vi "Graph ERD Read List.vi"(0 "GEA2 Reference In":refnum<k24>, 5 "GEA Inputs":T15={"Source"=229, "Destination"=35} {"Destination" format="%.0x"; "Source" format="%.0x"}, 7 "All_Bundled_Data_In":T1, 9 "ERD Graph Cntrl":T16={"ERD 3"={"ERD #"=0, "Data Type"=enum."uint16_t", "Scaler"=1}, "ERD 2"={"ERD #"=0, "Data Type"=enum."uint16_t", "Scaler"=1}, "ERD 1, ERD 2, & ERD3"={"ERD #"=0, "Data Type"=enum."uint16_t", "Scaler"=1}} {"ERD 1, ERD 2, & ERD3"."Scaler" min=1; "ERD 1, ERD 2, & ERD3"."ERD #" format="%.0x"; "ERD 2"."Scaler" min=1; "ERD 2"."ERD #" format="%.0x"; "ERD 3"."Scaler" min=1; "ERD 3"."ERD #" format="%.0x"}, 11 "Error In":errorcluster) -> (4 "GEA2 Reference Out":refnum<k24>, 6 "ERD Graph  Ind":T14, 10 "All_Bundled_Data_Brass Out":T1, 15 "Error Out":errorcluster)   [LabVIEW 2021]
uses:
  type defs/ERD_Graph_All_3.ctl
  type defs/ERD_Graph.ctl
  Common/LabVIEW GEA2 Toolkit/GEA3/type defs/Data Type.ctl
  D:/Common/LabVIEW GEA2 Toolkit/source/GEA3 DLL Source/GeaCommunication.dll
  Common/LabVIEW GEA2 Toolkit/source/GEA3 DLL Source/GeaCommunication.dll
  Common/LabVIEW GEA2 Toolkit/GEA3/type defs/Source_Destination.ctl
  type defs/All_Bundled_Data.ctl
  type defs/Version.ctl
  type defs/ERD_Always_Show.ctl
  type defs/Brass Matrix.ctl
  type defs/CSV_File_String_Arrays.ctl
  type defs/Redundant.ctl
  type defs/Algorithms.ctl
  type defs/ATC_Data.ctl
  type defs/Fault Table Array.ctl
  type defs/Fault_Table_Info.ctl
  Dryer Tool (Commercial 2)/JL Dryer Tool Support/type defs/ERD_RJ45.ctl
  Dryer Tool (Commercial 2)/JL Dryer Tool Support/type defs/ERD_Commercial_Laundry.ctl
  type defs/BootloaderVersion.ctl
  Common/LabVIEW GEA2 Toolkit/GEA3/type defs/ERD Read Data In.ctl
panel:
  # "Wet Load Size"
  # "Dry Load Size"
  # "OOB"
  # "Wet Load Size"
  # "Dry Load Size"
  # "OOB"
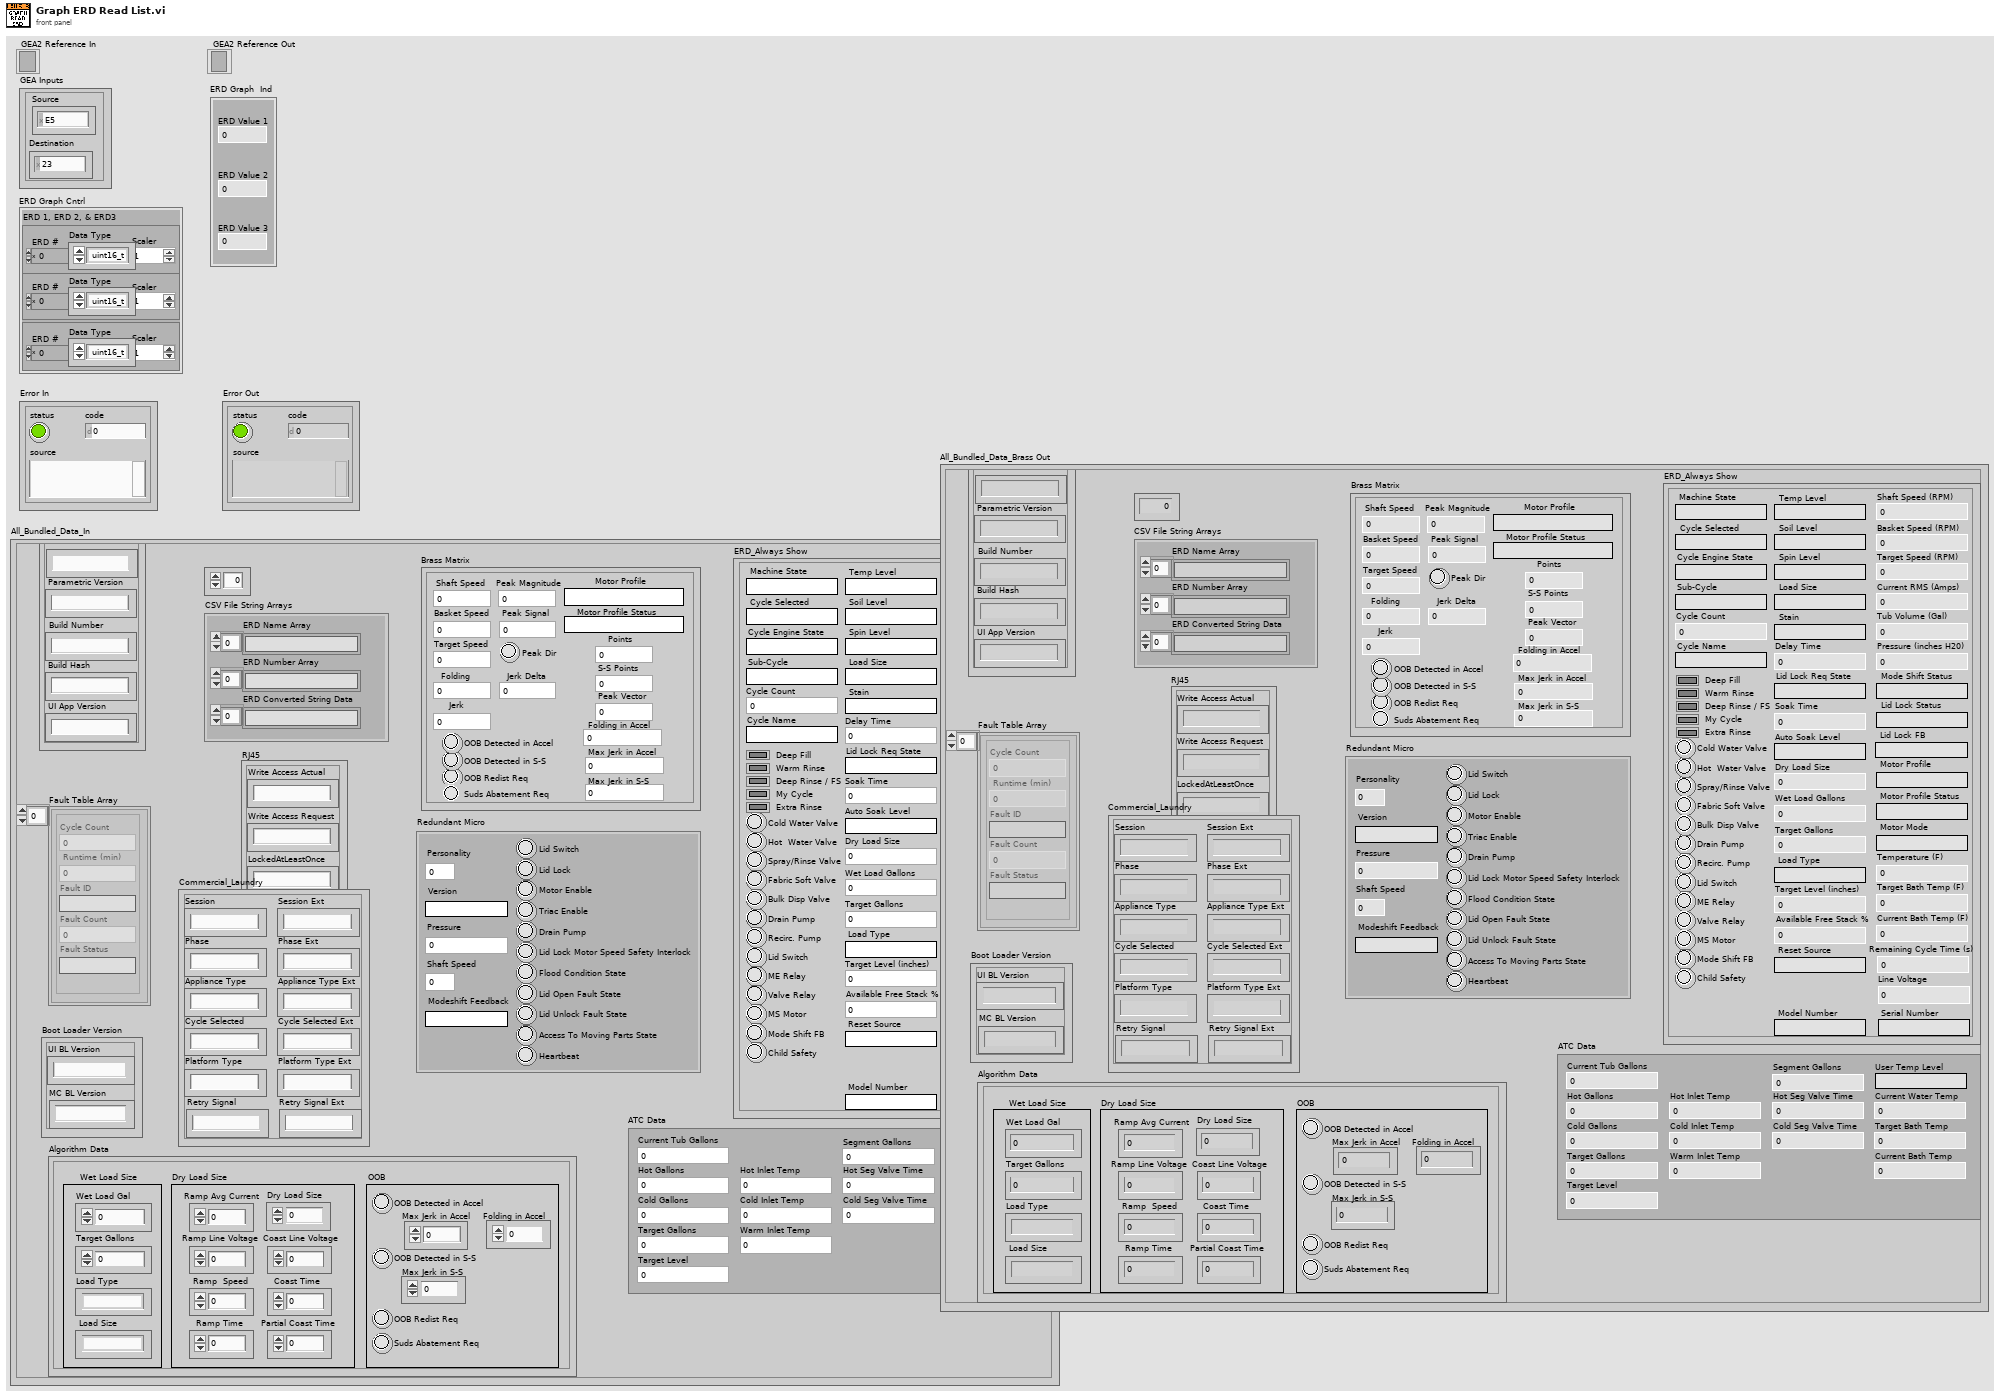
[diagram p1: front panel]
types:
  T1 = typedef "All_Bundled_Data.ctl" = cluster{"Software MC":T2, "ERD_Always Show":T3, "Personality Set":u8, "Brass Matrix":T4, "CSV File String Arrays":T5, "Redundant Micro":T6, "Algorithm Data":T7, "ATC Data":T8, "Fault Table Array ":T9, "RJ45":T11, "Commercial_Laundry":T12, "Boot Loader Version":T13}
  T2 = typedef "Version.ctl" = cluster{"Build Number":string, "Build Hash ":string, "Application Version":string, "Parametric Version":string, "UI App Version":string}
  T3 = typedef "ERD_Always_Show.ctl" = cluster{"Basket Speed (RPM)":u16, "Machine State":string, "Tub Volume (Gal)":dbl, "Pressure (inches H20)":dbl, "Lid Switch ":bool, "Current RMS (Amps)":dbl, "Cycle Selected":string, "Lid Lock Status":string, "Mode Shift Status":string, "Spray/Rinse Valve":bool, "Fabric Soft Valve":bool, "Drain Pump":bool, "Recirc. Pump":bool, "Cycle Engine State":string, "Hot  Water Valve":bool, "Cold Water Valve":bool, "Motor Profile":string, "Motor Profile Status":string, "Motor Mode":string, "ME Relay":bool, "Cycle Count":u32, "Deep Rinse / FS":bool, "My Cycle":bool, "Soil Level":string, "Spin Level":string, "Stain":string, "Temp Level":string, "Load Size":string, "Delay Time":u16, "Soak Time":u16, "Deep Fill":bool, "Warm Rinse":bool, "Auto Soak Level":string, "Extra Rinse":bool, "Wet Load Gallons":dbl, "Target Gallons":dbl, "Sub-Cycle":string, "Load Type":string, "Target Level (inches)":dbl, "Valve Relay":bool, "Dry Load Size":dbl, "Shaft Speed (RPM) ":u16, "MS Motor":bool, "Mode Shift FB":bool, "Target Bath Temp (F)":dbl, "Temperature (F)":dbl, "Current Bath Temp (F)":dbl, "Lid Lock FB":string, "Lid Lock Req State":string, "Remaining Cycle Time (s)":u32, "Available Free Stack %":u8, "Child Safety":bool, "Target Speed (RPM)":u16, "Reset Source":string, "Line Voltage":dbl, "Cycle Name":string, "Bulk Disp Valve":bool, "Model Number":string, "Serial Number":string}
  T4 = typedef "Brass Matrix.ctl" = cluster{"Shaft Speed":u16, "Folding":i32, "Jerk":i32, "Basket Speed":u16, "Target Speed":u16, "Peak Signal":u8, " Peak Magnitude":dbl, "Folding in Accel":i32, "Max Jerk in Accel":i32, "Max Jerk in S-S":i32, "Motor Profile Status":string, "Motor Profile":string, "OOB Redist Req":bool, "OOB Detected in S-S":bool, "OOB Detected in Accel":bool, "Suds Abatement Req ":bool, "Peak Dir":bool, "Peak Vector":dbl, "S-S Points":u8, "Points":u8, "Jerk Delta":i32}
  T5 = typedef "CSV_File_String_Arrays.ctl" = cluster{"ERD Number Array":string[], "ERD Name Array":string[], "ERD Converted String Data":string[]}
  T6 = typedef "Redundant.ctl" = cluster{"Version":string, "Personality":u8, "Pressure ":dbl, "Shaft Speed":u16, "Modeshift Feedback":string, "Lid Switch":bool, "Lid Lock":bool, "Triac Enable":bool, "Drain Pump":bool, "Lid Lock Motor Speed Safety Interlock":bool, "Flood Condition State":bool, "Lid Open Fault State":bool, "Access To Moving Parts State":bool, "Heartbeat":bool, "Motor Enable":bool, "Lid Unlock Fault State":bool}
  T7 = typedef "Algorithms.ctl" = cluster{"Wet Load Gal":dbl, "Target Gallons":dbl, "Load Type":string, "Load Size":string, "Coast Time":u16, "Ramp Time":u16, "Ramp  Speed":u16, "Ramp Avg Current":dbl, "OOB Redist Req":bool, "OOB Detected in S-S":bool, "Folding in Accel":i32, "Max Jerk in Accel":i32, "Max Jerk in S-S":i32, "OOB Detected in Accel":bool, "Partial Coast Time":u16, "Dry Load Size":dbl, "Ramp Line Voltage ":dbl, "Coast Line Voltage":dbl, "Suds Abatement Req ":bool}
  T8 = typedef "ATC_Data.ctl" = cluster{"Current Tub Gallons":dbl, "Hot Gallons":dbl, "Cold Gallons":dbl, "Target Gallons":dbl, "Current Water Temp":dbl, "Target Level":dbl, "Target Bath Temp":dbl, "Current Bath Temp ":dbl, "Cold Inlet Temp":dbl, "Hot Inlet Temp":dbl, "Warm Inlet Temp":dbl, "Hot Seg Valve Time":u16, "Cold Seg Valve Time ":u16, "User Temp Level":string, "Segment Gallons":dbl}
  T9 = typedef "Fault Table Array.ctl" = T10[]
  T10 = typedef "Fault_Table_Info.ctl" = cluster{"Cycle Count":u32, " Runtime (min) ":u32, "Fault Status":string, "Fault ID":string, "Fault Count":u16}
  T11 = typedef "ERD_RJ45.ctl" = cluster{"Write Access Actual":string, "Write Access Request":string, "LockedAtLeastOnce":string}
  T12 = typedef "ERD_Commercial_Laundry.ctl" = cluster{"Session":string, "Phase":string, "Appliance Type":string, "Cycle Selected":string, "Platform Type":string, "Retry Signal":string, "Session Ext":string, "Phase Ext":string, "Appliance Type Ext":string, "Cycle Selected Ext":string, "Platform Type Ext":string, "Retry Signal Ext":string}
  T13 = typedef "BootloaderVersion.ctl" = cluster{"UI BL Version":string, "MC BL Version":string}
  T14 = cluster{"ERD Value 1":dbl, "ERD Value 2":dbl, "ERD Value 3":dbl}
  T15 = typedef "Source_Destination.ctl" = cluster{"Source":u8, "Destination":u8}
  T16 = typedef "ERD_Graph_All_3.ctl" = cluster{"ERD 3":T17, "ERD 2":T17, "ERD 1, ERD 2, & ERD3":T17}
  T17 = typedef "ERD_Graph.ctl" = cluster{"ERD #":u16, "Data Type":T18, "Scaler":u32}
  T18 = typedef "Data Type.ctl" = enum16{"string", "boolean", "uint8_t", "uint16_t", "uint32_t", "uint64_t", "int8_t", "int16_t", "int32_t", "int64_t"}
  T19 = typedef "ERD Read Data In.ctl" = cluster{"ERD Number":u16, "Data Type":enum16{"string", "boolean", "uint8_t", "uint16_t", "uint32_t", "uint64_t", "int8_t", "int16_t", "int32_t", "int64_t"}}
  T20 = typedef "ERD Read Data Out.ctl" = cluster{"ERD Number":u16, "Data":string}
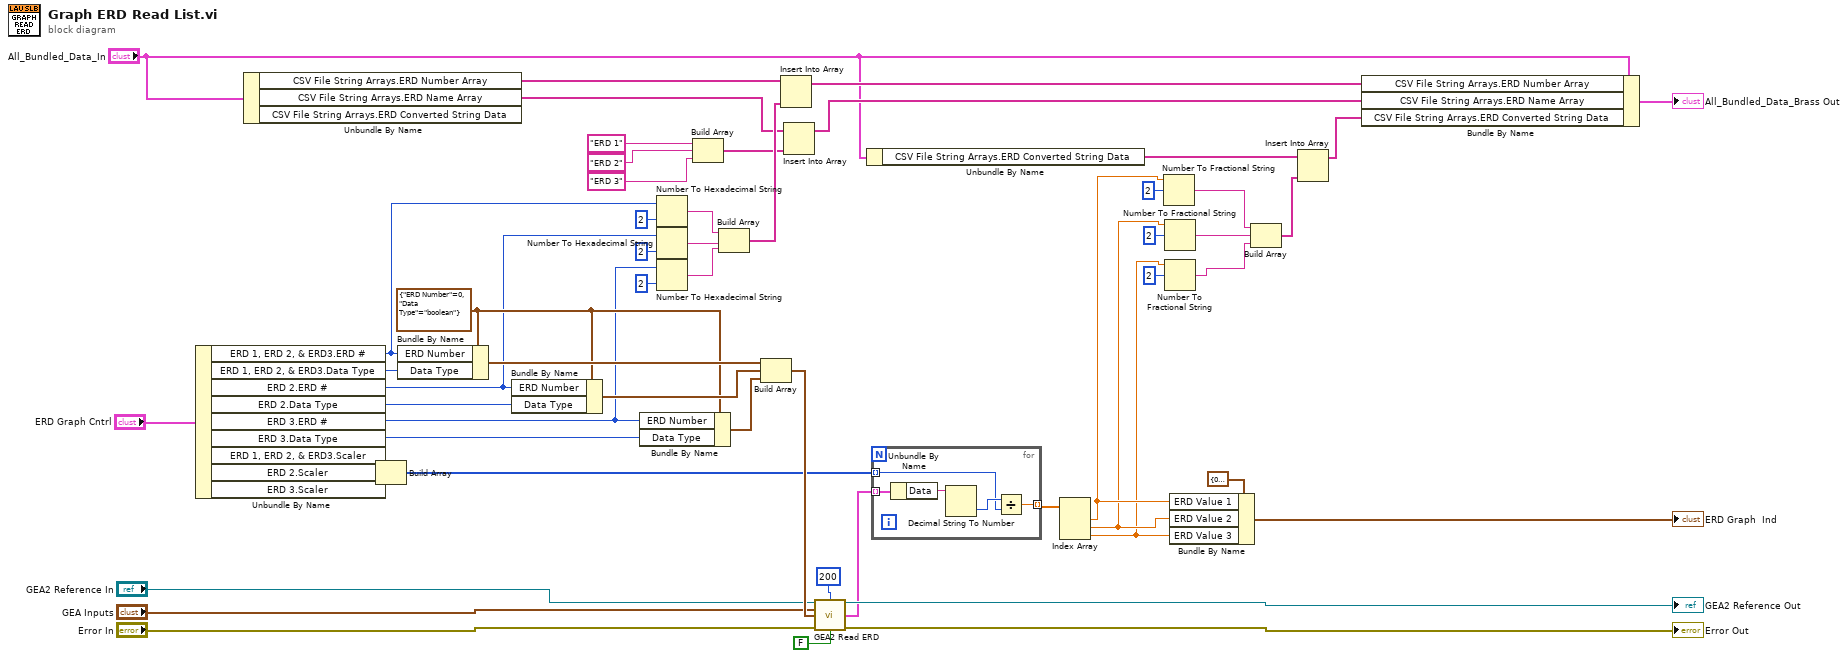
[diagram p0: block diagram]
diagram:
  w52 = T19 {"ERD Number"=0, "Data Type"=enum."boolean"} ("ERD Read Data In 2")
  n1 = Unbundle By Name("ERD Graph Cntrl") -> ("ERD 1, ERD 2, & ERD3.ERD #"=w29:u16, "ERD 1, ERD 2, & ERD3.Data Type"=w49:T18, "ERD 2.ERD #"=w28:u16, "ERD 2.Data Type"=w50:T18, "ERD 3.ERD #"=w27:u16, "ERD 3.Data Type"=w51:T18, "ERD 1, ERD 2, & ERD3.Scaler"=w42:u32, "ERD 2.Scaler"=w41:u32, "ERD 3.Scaler"=w40:u32)
  n2 = Unbundle By Name("All_Bundled_Data_In") -> ("CSV File String Arrays.ERD Number Array"=w22:string[], "CSV File String Arrays.ERD Name Array"=w19:string[])  [unwired: 1 out]
  n3 = Build Array(w42, w41, w40) -> (w39:u32[])
  n4 = Bundle By Name(cluster=w52, "ERD Number"=w29, "Data Type"=w49) -> (w53:T19)
  n5 = Bundle By Name(cluster=w52, "ERD Number"=w28, "Data Type"=w50) -> (w54:T19)
  n6 = Bundle By Name(cluster=w52, "ERD Number"=w27, "Data Type"=w51) -> (w55:T19)
  n7 = Number To Hexadecimal String(1:i16 2 ("width (-)"), 2:w29) -> (0:w26:string)
  n8 = Number To Hexadecimal String(1:i16 2 ("width (-)"), 2:w28) -> (0:w25:string)
  n9 = Number To Hexadecimal String(1:i16 2 ("width (-)"), 2:w27) -> (0:w24:string)
  n10 = Build Array("ERD 1", "ERD 2", "ERD 3") -> (w18:string[])
  n11 = Build Array(w26, w25, w24) -> (w23:string[])
  n12 = Build Array(w53, w54, w55) -> (w48:T19[])
  n13 = Insert Into Array(array=w22, new element=w23) -> (w20:string[])  [unwired: 1 in]
  n14 = Insert Into Array(array=w19, new element=w18) -> (w14:string[])  [unwired: 1 in]
  n15 = call "GEA2 Read ERD.vi"("GEA2 Reference In"="GEA2 Reference In", "Read Timeout (ms)"=u32 200, "GEA Inputs"="GEA Inputs", "Read ERD List"=w48, "Error In"="Error In", "Verify ERD Response?"=FALSE) -> ("GEA2 Reference Out"=→"GEA2 Reference Out":refnum<k24>, "ERD Data Out"=w38:T20[], "Error Out"=→"Error Out":errorcluster)  [unwired: 6 in, 1 out]
  n16 = Unbundle By Name("All_Bundled_Data_In") -> ("CSV File String Arrays.ERD Converted String Data"=w3:string[])
  n17 = for {
    tunnel: w39 -> [w58] mode=indexing
    tunnel: w38 -> [w61] mode=indexing
    tunnel: [w57] -> w37 mode=indexing
    n18 = Unbundle By Name(w61) -> ("Data"=w60:string)
    n19 = Decimal String To Number(string=w60) -> (number=w59:i32)  [unwired: 2 in, 1 out]
    n20 = Divide(x=w59, y=w58) -> (x/y=w57:dbl)
  }
  n21 = Index Array(array=w37) -> (element #1=w13:dbl, element #2=w9:dbl, element #3=w8:dbl)  [unwired: 3 in]
  n22 = Number To Fractional String(number=w13, width (-)=i16 2) -> (F-format string=w7:string)  [unwired: 2 in]
  n23 = Number To Fractional String(number=w9, width (-)=i16 2) -> (F-format string=w6:string)  [unwired: 2 in]
  n24 = Number To Fractional String(number=w8, width (-)=i16 2) -> (F-format string=w5:string)  [unwired: 2 in]
  n25 = Bundle By Name(cluster=T14 {"ERD Value 1"=0.0, "ERD Value 2"=0.0, "ERD Value 3"=0.0} ("ERD Graph  Ind"), "ERD Value 1"=w13, "ERD Value 2"=w9, "ERD Value 3"=w8) -> (→"ERD Graph  Ind":T14)
  n26 = Build Array(w7, w6, w5) -> (w2:string[])
  n27 = Insert Into Array(array=w3, new element=w2) -> (w1:string[])  [unwired: 1 in]
  n28 = Bundle By Name(cluster="All_Bundled_Data_In", "CSV File String Arrays.ERD Number Array"=w20, "CSV File String Arrays.ERD Name Array"=w14, "CSV File String Arrays.ERD Converted String Data"=w1) -> (→"All_Bundled_Data_Brass Out":T1)
